vi "Axsun_module.vi"() -> ()   [LabVIEW 2018]
uses:
  cluster_Axsun.ctl
  Queue Manager Actions.ctl
  MessagePacket.ctl
  QueueNames.ctl
  C:/AlazarTech/ATS-SDK/7.2.0/Samples_LabVIEW/ATS9350/Dual Port/stephan/AxsunOCTControl.dll
  AxsunOCTControl.dll
panel:
  in  "clock delay":u32
  in  "GetStatus":bool
  in  "LaserOnTime":bool
  out "output cluster":T1
  out "GUI error":errorcluster
  in  "Source current OFF":bool
  in  "Source current ON":bool
  in  "stop":bool
  in  "Laser OFF":bool
  in  "Laser ON":bool
  out "processor error":errorcluster
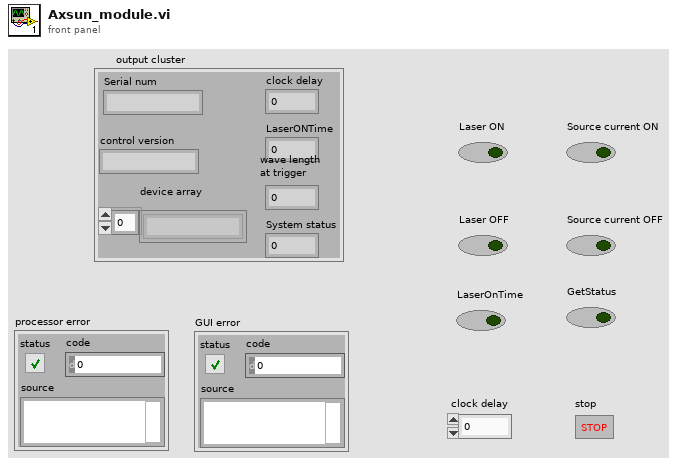
[diagram p1: front panel]
types:
  T1 = typedef "cluster_Axsun.ctl" = cluster{"device array":string[], "control version":string, "Serial num":string, "LaserONTime":i32, "wave length\nat trigger":dbl, "System status":dbl, "clock delay":u32}
  T2 = typedef "MessagePacket.ctl" = cluster{"Message":string, "Parameter":variant}
  T3 = typedef "Queue Manager Actions.ctl" = enum16{"Init", "Enqueue", "Enqueue All", "Preview Queue", "Dequeue", "Get Status", "Flush Queue", "Flush All Queues", "Release All Queues", "Release Queue", "Enqueue at Opposite End"}
  T4 = typedef "QueueNames.ctl" = enum16{"Main GUI", "Main Scan Processor", "Axsun GUI", "Axsun processor", "Main Display", "Main Table Stage GUI", "Main Table Stage Proc.", "Scan Engine", "Vibratome GUI", "Vibratome Processor", "Slice Engine"}
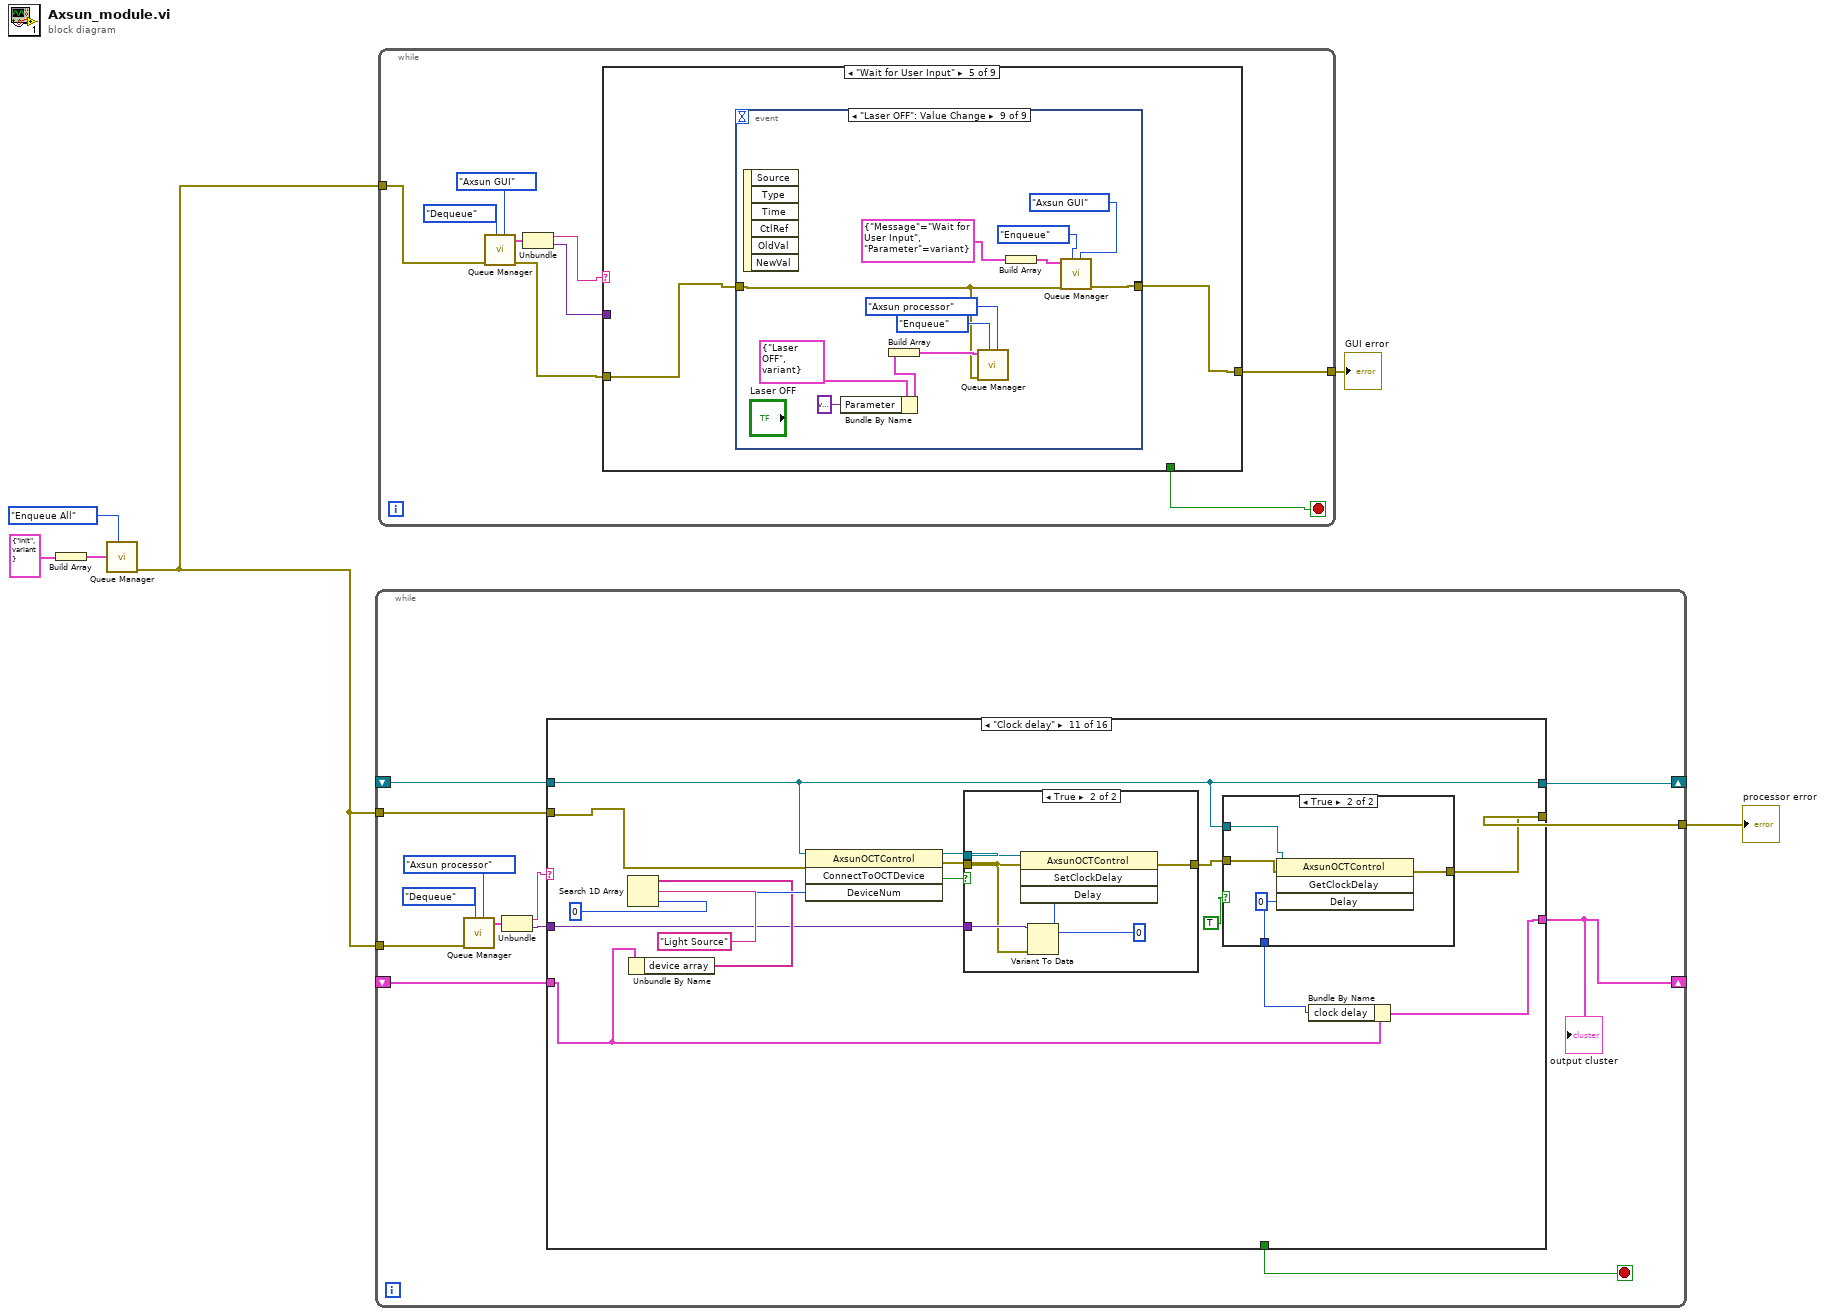
[diagram p0: block diagram]
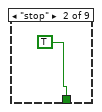
[diagram p3: hidden frame]
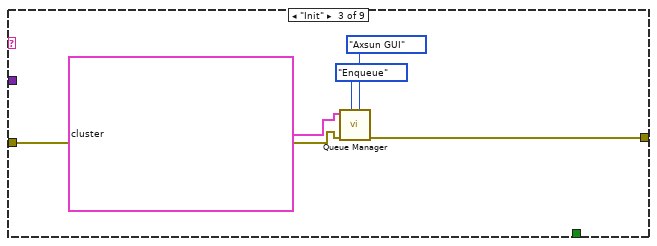
[diagram p4: hidden frame]
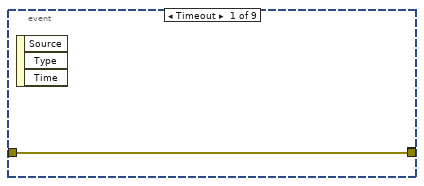
[diagram p6: hidden frame]
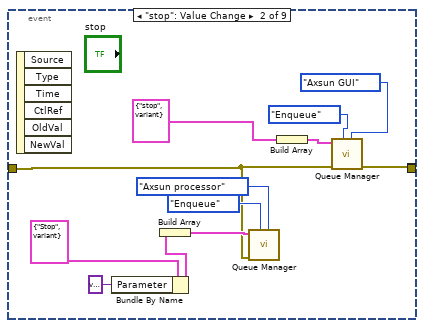
[diagram p7: hidden frame]
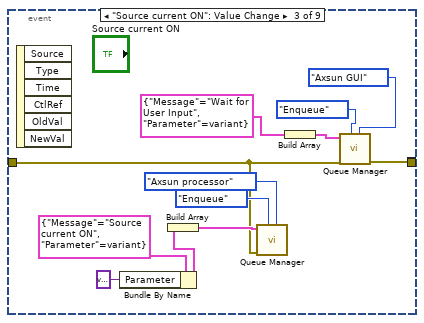
[diagram p8: hidden frame]
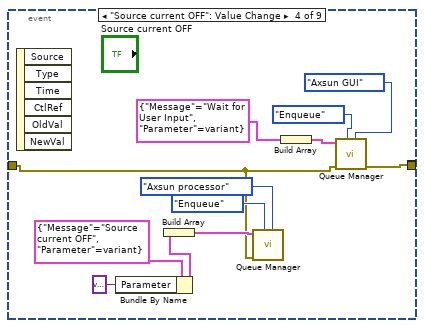
[diagram p9: hidden frame]
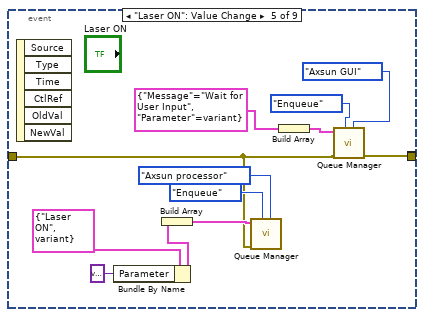
[diagram p10: hidden frame]
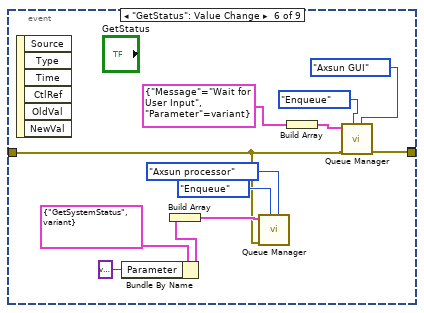
[diagram p11: hidden frame]
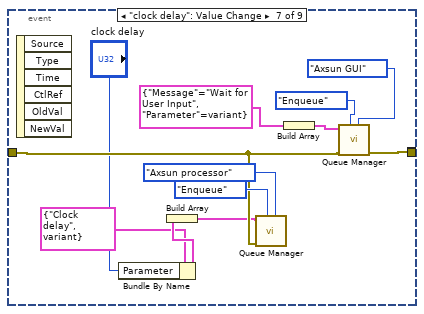
[diagram p12: hidden frame]
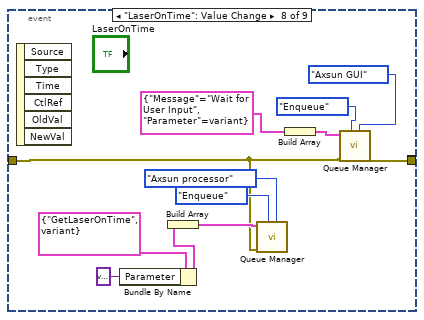
[diagram p13: hidden frame]
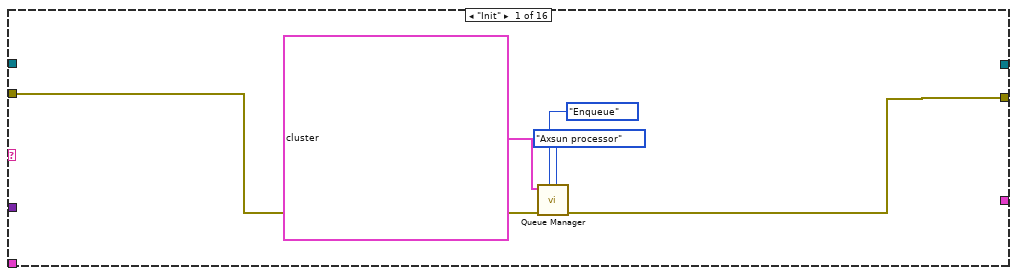
[diagram p18: hidden frame]
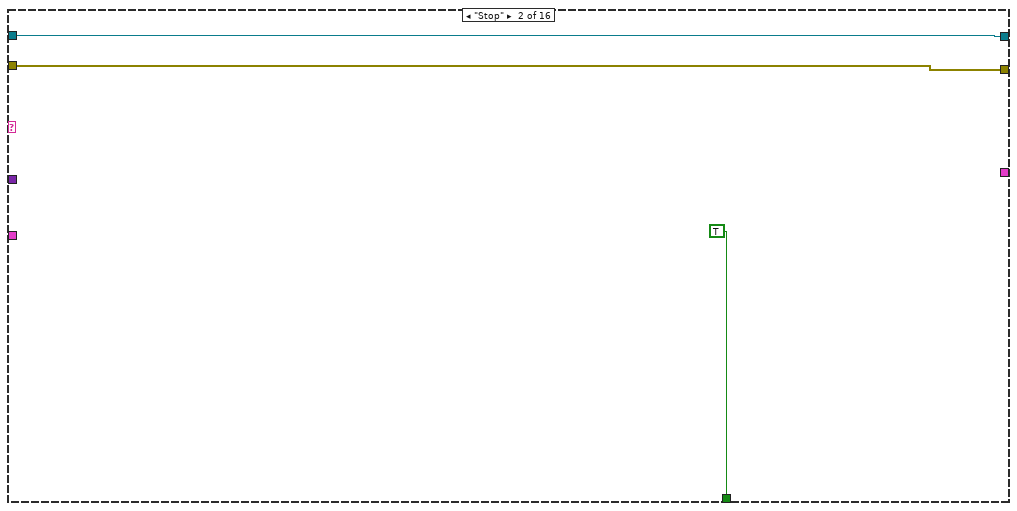
[diagram p19: hidden frame]
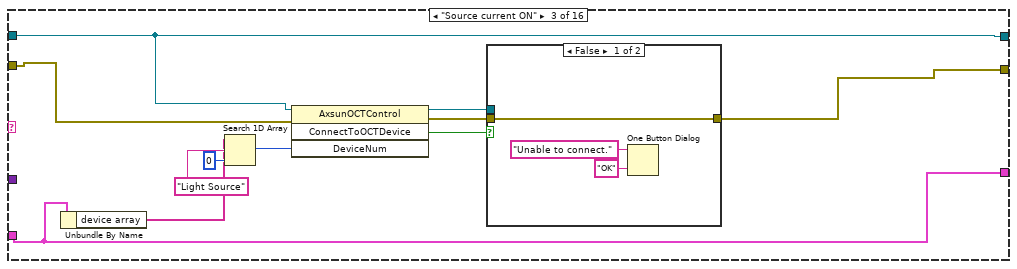
[diagram p20: hidden frame]
diagram:
  n1 = Build Array(T2 {"Message"="Init", "Parameter"=variant} ("Message Packet [In]")) -> (w4:T2[])
  n2 = call "Queue Manager.vi"("Action"=Queue_Manager_Actions."Enqueue All", "Message Packet Array"=w4) -> ("Error Out"=w2:errorcluster)  [unwired: 7 in, 2 out]
  n3 = while {
    shift-right: [w7] -> _
    shift-left: _ -> [w8]
    tunnel: w2 -> [w15]
    shift-right: [w9] -> _
    shift-left: _ -> [w12]
    tunnel: [w11] -> w3
    tunnel: w2 -> [w10]
    stop <- w14 stop-if-true
    n4 = call "Queue Manager.vi"("Queue Name"=QueueNames."Axsun processor", "Action"=Queue_Manager_Actions."Dequeue", "Error In"=w10) -> ("Message Packet [Out]"=w17:T2)  [unwired: 6 in, 2 out]
    n5 = Unbundle(w17) -> ("Message"=w13:string, "Parameter"=w16:variant)
    n6 = case shown="\"Clock delay\"" w13 {
      tunnel: w16 -> [_ _ _ _ _ _ _ _ _ _ w168 _ _ _ _ _]
      tunnel: w15 -> [w24 w26 w32 w48 w64 w69 w86 w106 w125 w146 w169 w198 w216 w223 w244 _]
      tunnel: [_ TRUE _ _ _ _ _ _ _ _ _ _ _ _ _ _] -> w14
      tunnel: [w20 w26 w31 w49 w64 w67 w82 w105 w124 w145 w165 w197 w215 w222 w243 w261] -> w11
      tunnel: [_ _ w30 w47 w63 w66 w75 w104 w123 w143 w163 w196 w213 w218 w240 w260] -> w9
      tunnel: w12 -> [_ _ w30 w47 w63 w66 _ w104 w121 w142 w164 w196 w214 w220 w241 w260]
      tunnel: [_ w25 w28 w45 w62 w65 w72 w102 w119 w140 w161 w194 w211 w217 w239 w259] -> w7
      tunnel: w8 -> [_ w25 w28 w45 w62 w65 w72 w102 w119 w140 w161 w194 w211 w217 w239 _]
      frame "Init" {
        n7 = call "Queue Manager.vi"("Queue Name"=QueueNames."Axsun processor", "Action"=Queue_Manager_Actions."Enqueue", "Error In"=w24, "Message Packet Array"=T2[] [{"Message"="Create handle", "Parameter"=variant}, {"Message"="Start Network Control Interface", "Parameter"=variant}, {"Message"="Get laser handle", "Parameter"=variant}, {"Message"="GetControlVersion", "Parameter"=variant}, {"Message"="GetSerialNum", "Parameter"=variant}, {"Message"="GetSystemStatus", "Parameter"=variant}, {"Message"="GetWaveLengthAtSweptTrigger", "Parameter"=variant}, {"Message"="GetLaserOnTime\nGetLaserOnTime", "Parameter"=variant}]) -> ("Error Out"=w20:errorcluster)  [unwired: 5 in, 2 out]
      }
      frame "Stop" {
      }
      frame "Source current ON" {
        n8 = Unbundle By Name(w30) -> ("device array"=w29:string[])
        n9 = Search 1D Array(1D array=w29, element="Light Source", start index (0)=0) -> (index of element=w36:i32)
        n10 = invoke class="AxsunOCTControl" method="ConnectToOCTDevice"(reference=w28, error in=w32, "DeviceNum"=w36) -> (reference out=w35:refnum<k24>, error out=w34:errorcluster, "ConnectToOCTDevice"=w33:bool)  [unwired: 1 in, 1 out]
        n11 = case shown="False" w33 {
          tunnel: w35 -> [_ w44]
          tunnel: w34 -> [w41 w43]
          tunnel: [w41 w42] -> w31
          frame False {
            n12 = One Button Dialog(message="Unable to connect.", button name ("OK")="OK") -> ()  [unwired: 1 out]
          }
          frame True {
            n13 = invoke class="AxsunOCTControl" method="SourceCurrentOn"(reference=w44, error in=w43) -> (error out=w42:errorcluster)  [unwired: 1 in, 2 out]
          }
        }
      }
      frame "Source current OFF" {
        n14 = Unbundle By Name(w47) -> ("device array"=w46:string[])
        n15 = Search 1D Array(1D array=w46, element="Light Source", start index (0)=0) -> (index of element=w53:i32)
        n16 = invoke class="AxsunOCTControl" method="ConnectToOCTDevice"(reference=w45, error in=w48, "DeviceNum"=w53) -> (reference out=w52:refnum<k24>, error out=w51:errorcluster, "ConnectToOCTDevice"=w50:bool)  [unwired: 1 in, 1 out]
        n17 = case shown="True" w50 {
          tunnel: w52 -> [_ w61]
          tunnel: w51 -> [w58 w60]
          tunnel: [w58 w59] -> w49
          frame False {
            n18 = One Button Dialog(message="Unable to connect.", button name ("OK")="OK") -> ()  [unwired: 1 out]
          }
          frame True {
            # "Turn laser emission ON"
            n19 = invoke class="AxsunOCTControl" method="SourceCurrentOff"(reference=w61, error in=w60) -> (error out=w59:errorcluster)  [unwired: 1 in, 2 out]
          }
        }
      }
      frame Default {
      }
      frame "Start Network Control Interface" {
        n20 = invoke class="AxsunOCTControl" method="StartNetworkControlInterface"(reference=w65, error in=w69) -> (error out=w68:errorcluster)  [unwired: 1 in, 2 out]
        n21 = flat-sequence {
          tunnel: w68 -> [w70]
          tunnel: [w70] -> w67
          frame #0 {
            n22 = Wait (ms)(milliseconds to wait=2000) -> ()  [unwired: 1 out]
          }
        }
      }
      frame "Get laser handle" {
        n23 = invoke class="AxsunOCTControl" method="GetNumberOfOCTDevicesPresent"(reference=w72, error in=w86) -> (reference out=w85:refnum<k24>, error out=w83:errorcluster, "GetNumberOfOCTDevicesPresent"=w84:i32)  [unwired: 1 in]
        n24 = for {
          N: w84 -> [_]
          tunnel: w85 -> [w92]
          tunnel: w83 -> [w91]
          tunnel: [w87] -> w77 mode=indexing
          tunnel: [w89] -> w82
          tunnel: [w88] -> _ mode=indexing
          i -> [w90]
          n25 = invoke class="AxsunOCTControl" method="ConnectToOCTDevice"(reference=w92, error in=w91, "DeviceNum"=w90) -> (reference out=w96:refnum<k24>, error out=w95:errorcluster)  [unwired: 1 in, 2 out]
          n26 = stacked-sequence {
            tunnel: w96 -> [w101]
            tunnel: [w101] -> w94
            tunnel: w95 -> [w100]
            tunnel: [w100] -> w93
            frame #0 {
              n27 = Wait (ms)(milliseconds to wait=u32 20) -> ()  [unwired: 1 out]
            }
          }
          n28 = invoke class="AxsunOCTControl" method="GetSystemType"(reference=w94, error in=w93, "SystemType"=u32 0, "SystemTypeString"="") -> (reference out=w88:refnum<k24>, error out=w89:errorcluster, "SystemTypeString"=w87:string)  [unwired: 1 in, 2 out]
        }
        n29 = Bundle By Name(cluster=T1 {"device array"=[], "control version"="", "Serial num"="", "LaserONTime"=0, "wave length\nat trigger"=0.0, "System status"=0.0, "clock delay"=0} ("output cluster"), "device array"=w77, "control version"="GetControlVersion", "Serial num"="''", "LaserONTime"=0, "wave length\nat trigger"=0.0, "System status"=0.0 ("Status"), "clock delay"=u32 0) -> (w75:T1)
      }
      frame "Laser ON" {
        n30 = Unbundle By Name(w104) -> ("device array"=w103:string[])
        n31 = Search 1D Array(1D array=w103, element="Light Source", start index (0)=0) -> (index of element=w110:i32)
        n32 = invoke class="AxsunOCTControl" method="ConnectToOCTDevice"(reference=w102, error in=w106, "DeviceNum"=w110) -> (reference out=w109:refnum<k24>, error out=w108:errorcluster, "ConnectToOCTDevice"=w107:bool)  [unwired: 1 in, 1 out]
        n33 = case shown="True" w107 {
          tunnel: w109 -> [_ w118]
          tunnel: w108 -> [w115 w117]
          tunnel: [w115 w116] -> w105
          frame False {
            n34 = One Button Dialog(message="Unable to .", button name ("OK")="OK") -> ()  [unwired: 1 out]
          }
          frame True {
            # "Turn laser emission ON"
            n35 = invoke class="AxsunOCTControl" method="StartScan"(reference=w118, error in=w117) -> (error out=w116:errorcluster)  [unwired: 1 in, 2 out]
          }
        }
      }
      frame "GetWaveLengthAtSweptTrigger" {
        n36 = Unbundle By Name(w121) -> ("device array"=w120:string[])
        n37 = Search 1D Array(1D array=w120, element="Light Source", start index (0)=0) -> (index of element=w129:i32)
        n38 = invoke class="AxsunOCTControl" method="ConnectToOCTDevice"(reference=w119, error in=w125, "DeviceNum"=w129) -> (reference out=w128:refnum<k24>, error out=w127:errorcluster, "ConnectToOCTDevice"=w126:bool)  [unwired: 1 in, 1 out]
        n39 = case shown="False" w126 {
          tunnel: w128 -> [_ w139]
          tunnel: w127 -> [w134 w138]
          tunnel: [w134 w137] -> w124
          tunnel: [_ w135] -> w122
          frame False {
            n40 = One Button Dialog(message="Unable to .", button name ("OK")="OK") -> ()  [unwired: 1 out]
          }
          frame True {
            # "Turn laser emission ON"
            n41 = invoke class="AxsunOCTControl" method="GetWavelengthAtSweepTrigger"(reference=w139, error in=w138, "Wavelength"=0.0) -> (error out=w137:errorcluster, "Wavelength"=w135:dbl)  [unwired: 1 in, 2 out]
          }
        }
        n42 = Bundle(cluster=w121, "LaserONTime"=w122) -> (w123:T1)  [unwired: 6 in]
      }
      frame "GetLaserOnTime" {
        # "Make active board = laser"
        n43 = Unbundle By Name(w142) -> ("device array"=w141:string[])
        n44 = Search 1D Array(1D array=w141, element="Light Source", start index (0)=0) -> (index of element=w152:i32)
        n45 = invoke class="AxsunOCTControl" method="ConnectToOCTDevice"(reference=w140, error in=w146, "DeviceNum"=w152) -> (reference out=w148:refnum<k24>, error out=w149:errorcluster, "ConnectToOCTDevice"=w147:bool)  [unwired: 1 in, 1 out]
        n46 = case shown="False" w147 {
          tunnel: w149 -> [w155 w159]
          tunnel: w148 -> [_ w160]
          tunnel: [w155 w158] -> w145
          tunnel: [_ w156] -> w144
          frame False {
            n47 = One Button Dialog(message="Unable to connect.", button name ("OK")="OK") -> ()  [unwired: 1 out]
          }
          frame True {
            n48 = invoke class="AxsunOCTControl" method="GetLaserOnTime"(reference=w160, error in=w159, "LaserOnTimeSeconds"=u32 0) -> (error out=w158:errorcluster, "LaserOnTimeSeconds"=w156:u32)  [unwired: 1 in, 2 out]
          }
        }
        n49 = Bundle(cluster=w142, "LaserONTime"=w144) -> (w143:T1)  [unwired: 6 in]
      }
      frame "Clock delay" {
        n50 = Unbundle By Name(w164) -> ("device array"=w170:string[])
        n51 = Search 1D Array(1D array=w170, element="Light Source", start index (0)=0) -> (index of element=w174:i32)
        n52 = invoke class="AxsunOCTControl" method="ConnectToOCTDevice"(reference=w161, error in=w169, "DeviceNum"=w174) -> (reference out=w173:refnum<k24>, error out=w172:errorcluster, "ConnectToOCTDevice"=w171:bool)  [unwired: 1 in, 1 out]
        n53 = case shown="True" w171 {
          tunnel: w173 -> [_ w193]
          tunnel: w172 -> [w187 w189]
          tunnel: [w187 w188] -> w167
          tunnel: w168 -> [_ w192]
          frame False {
            n54 = One Button Dialog(message="Unable to connect.", button name ("OK")="OK") -> ()  [unwired: 1 out]
          }
          frame True {
            n55 = Variant To Data(error in=w189, type=u32 0 ("Delay"), Variant=w192) -> (data=w190:u32)  [unwired: 1 out]
            n56 = invoke class="AxsunOCTControl" method="SetClockDelay"(reference=w193, error in=w189, "Delay"=w190) -> (error out=w188:errorcluster)  [unwired: 1 in, 3 out]
          }
        }
        n57 = case shown="True" TRUE {
          tunnel: w167 -> [w179 w184]
          tunnel: [w179 w183] -> w165
          tunnel: [_ w181] -> w162
          tunnel: w161 -> [_ w180]
          frame False {
            n58 = One Button Dialog(message="Unable to connect.", button name ("OK")="OK") -> ()  [unwired: 1 out]
          }
          frame True {
            n59 = invoke class="AxsunOCTControl" method="GetClockDelay"(reference=w180, error in=w184, "Delay"=u32 0) -> (error out=w183:errorcluster, "Delay"=w181:u32)  [unwired: 1 in, 2 out]
          }
        }
        n60 = Bundle By Name(cluster=w164, "clock delay"=w162) -> (w163:T1)
      }
      frame "Laser OFF" {
        # "Make active board = laser"
        n61 = Unbundle By Name(w196) -> ("device array"=w195:string[])
        n62 = Search 1D Array(1D array=w195, element="Light Source", start index (0)=0) -> (index of element=w202:i32)
        n63 = invoke class="AxsunOCTControl" method="ConnectToOCTDevice"(reference=w194, error in=w198, "DeviceNum"=w202) -> (reference out=w201:refnum<k24>, error out=w200:errorcluster, "ConnectToOCTDevice"=w199:bool)  [unwired: 1 in, 1 out]
        n64 = case shown="True" w199 {
          tunnel: w201 -> [_ w210]
          tunnel: w200 -> [w207 w209]
          tunnel: [w207 w208] -> w197
          frame False {
            n65 = One Button Dialog(message="Unable to connect.", button name ("OK")="OK") -> ()  [unwired: 1 out]
          }
          frame True {
            # "Turn laser emission ON"
            n66 = invoke class="AxsunOCTControl" method="StopScan"(reference=w210, error in=w209) -> (error out=w208:errorcluster)  [unwired: 1 in, 2 out]
          }
        }
      }
      frame "GetControlVersion" {
        n67 = invoke class="AxsunOCTControl" method="GetControlVersion"(reference=w211, error in=w216) -> (error out=w215:errorcluster, "GetControlVersion"=w212:string)  [unwired: 1 in, 1 out]
        n68 = Bundle By Name(cluster=w214, "control version"=w212) -> (w213:T1)
      }
      frame "GetSerialNum" {
        n69 = Unbundle By Name(w220) -> ("device array"=w221:string[])
        n70 = Search 1D Array(1D array=w221, element="Light Source", start index (0)=0) -> (index of element=w227:i32)
        n71 = invoke class="AxsunOCTControl" method="ConnectToOCTDevice"(reference=w217, error in=w223, "DeviceNum"=w227) -> (reference out=w226:refnum<k24>, error out=w225:errorcluster, "ConnectToOCTDevice"=w224:bool)  [unwired: 1 in, 1 out]
        n72 = case shown="True" w224 {
          tunnel: w226 -> [_ w237]
          tunnel: w225 -> [w232 w236]
          tunnel: [w232 w235] -> w222
          tunnel: [_ w233] -> w219
          frame False {
            n73 = One Button Dialog(message="Unable to connect.", button name ("OK")="OK") -> ()  [unwired: 1 out]
          }
          frame True {
            n74 = invoke class="AxsunOCTControl" method="GetSerialNum"(reference=w237, error in=w236, "SerialNum"="") -> (error out=w235:errorcluster, "SerialNum"=w233:string)  [unwired: 1 in, 2 out]
          }
        }
        n75 = Bundle By Name(cluster=w220, "Serial num"=w219) -> (w218:T1)
      }
      frame "GetSystemStatus" {
        # "Make active board = laser"
        n76 = Unbundle By Name(w241) -> ("device array"=w242:string[])
        n77 = Search 1D Array(1D array=w242, element="Light Source", start index (0)=0) -> (index of element=w249:i32)
        n78 = invoke class="AxsunOCTControl" method="ConnectToOCTDevice"(reference=w239, error in=w244, "DeviceNum"=w249) -> (error out=w245:errorcluster, "ConnectToOCTDevice"=w246:bool)  [unwired: 1 in, 2 out]
        n79 = case shown="True" w246 {
          tunnel: w245 -> [w252 w258]
          tunnel: [w252 w255] -> w243
          tunnel: [_ w254] -> w238
          tunnel: w239 -> [_ w253]
          frame False {
            n80 = One Button Dialog(message="Unable to connect.", button name ("OK")="OK") -> ()  [unwired: 1 out]
          }
          frame True {
            n81 = invoke class="AxsunOCTControl" method="GetSystemStatus"(reference=w253, error in=w258, "StatusArray"=u32[] [], "StatusWordsReturned"=u32 0) -> (error out=w255:errorcluster, "StatusWordsReturned"=w254:u32)  [unwired: 1 in, 3 out]
          }
        }
        n82 = Bundle By Name(cluster=w241, "System status"=w238) -> (w240:T1)
      }
      frame "Create handle" {
        n83 = constructor class="AxsunOCTControl"() -> (reference out=w259:refnum<k24>, error out=w261:errorcluster)  [unwired: 3 in, 1 out]
      }
    }
    "output cluster" <- w9
  }
  "processor error" <- w3
  n84 = while {
    tunnel: w2 -> [w267]
    tunnel: [w263] -> w1
    stop <- w262 stop-if-true
    n85 = call "Queue Manager.vi"("Queue Name"=QueueNames."Axsun GUI", "Action"=Queue_Manager_Actions."Dequeue", "Error In"=w267) -> ("Error Out"=w264:errorcluster, "Message Packet [Out]"=w268:T2)  [unwired: 6 in, 1 out]
    n86 = Unbundle(w268) -> ("Message"=w266:string, "Parameter"=w265:variant)
    n87 = case shown="\"Wait for User Input\"" w266 {
      tunnel: w265 -> [_ _ _ _ _ _ _ _ _]
      tunnel: w264 -> [w271 _ w277 w278 w280 w378 w379 w380 w381]
      tunnel: [w271 _ w274 w278 w279 w378 w379 w380 w381] -> w263
      tunnel: [_ TRUE _ _ _ _ _ _ _] -> w262
      frame "False", Default {
      }
      frame "stop" {
      }
      frame "Init" {
        n88 = call "Queue Manager.vi"("Queue Name"=QueueNames."Axsun GUI", "Action"=Queue_Manager_Actions."Enqueue", "Error In"=w277, "Message Packet Array"=T2[] [{"Message"="Wait for Complete", "Parameter"=variant}, {"Message"="Set Front Panel", "Parameter"=variant}, {"Message"="Load User Settings", "Parameter"=variant}, {"Message"="Configure Hardware", "Parameter"=variant}, {"Message"="Configure Hardware", "Parameter"=variant}, {"Message"="Wait for User Input", "Parameter"=variant}]) -> ("Error Out"=w274:errorcluster)  [unwired: 5 in, 2 out]
      }
      frame "Set Front Panel" {
      }
      frame "Wait for User Input" {
        n89 = event shown="[8] \"Laser OFF\": Value Change" {
          selector: _ -> [_ _ _ _ _ _ _ _ _]
          dyn-events: _ -> [_ _ _ _ _ _ _ _ _]
          timeout: _ -> [_ _ _ _ _ _ _ _ _]
          tunnel: w280 -> [w281 w282 w294 w306 w318 w331 w346 w355 w366]
          tunnel: [_ w283 w295 w307 w322 w330 w345 w354 w368] -> w279
          tunnel: [w281 _ _ _ _ _ _ _ _] -> _
          event Timeout {
            n90 = event-data() -> ()  [unwired: 1 in, 3 out]
          }
          event "stop": Value Change {
            n91 = event-data() -> ()  [unwired: 1 in, 6 out]
            n92 = Bundle By Name(cluster=T2 {"Message"="Stop", "Parameter"=variant} ("Message Packet [In]"), "Parameter"=variant) -> (w289:T2)
            n93 = Build Array(w289) -> (w286:T2[])
            n94 = call "Queue Manager.vi"("Queue Name"=QueueNames."Axsun processor", "Action"=Queue_Manager_Actions."Enqueue", "Error In"=w282, "Message Packet Array"=w286) -> ()  [unwired: 5 in, 3 out]
            n95 = Build Array(T2 {"Message"="stop", "Parameter"=variant} ("Message Packet [In]")) -> (w293:T2[])
            n96 = call "Queue Manager.vi"("Queue Name"=QueueNames."Axsun GUI", "Action"=Queue_Manager_Actions."Enqueue", "Error In"=w282, "Message Packet Array"=w293) -> ("Error Out"=w283:errorcluster)  [unwired: 5 in, 2 out]
          }
          event "Source current ON": Value Change {
            n97 = event-data() -> ()  [unwired: 1 in, 6 out]
            n98 = Bundle By Name(cluster=T2 {"Message"="Source current ON", "Parameter"=variant} ("Message Packet [In]"), "Parameter"=variant) -> (w301:T2)
            n99 = Build Array(w301) -> (w298:T2[])
            n100 = call "Queue Manager.vi"("Queue Name"=QueueNames."Axsun processor", "Action"=Queue_Manager_Actions."Enqueue", "Error In"=w294, "Message Packet Array"=w298) -> ()  [unwired: 5 in, 3 out]
            n101 = Build Array(T2 {"Message"="Wait for User Input", "Parameter"=variant} ("Message Packet [In]")) -> (w305:T2[])
            n102 = call "Queue Manager.vi"("Queue Name"=QueueNames."Axsun GUI", "Action"=Queue_Manager_Actions."Enqueue", "Error In"=w294, "Message Packet Array"=w305) -> ("Error Out"=w295:errorcluster)  [unwired: 5 in, 2 out]
          }
          event "Source current OFF": Value Change {
            n103 = event-data() -> ()  [unwired: 1 in, 6 out]
            n104 = Bundle By Name(cluster=T2 {"Message"="Source current OFF", "Parameter"=variant} ("Message Packet [In]"), "Parameter"=variant) -> (w313:T2)
            n105 = Build Array(w313) -> (w310:T2[])
            n106 = call "Queue Manager.vi"("Queue Name"=QueueNames."Axsun processor", "Action"=Queue_Manager_Actions."Enqueue", "Error In"=w306, "Message Packet Array"=w310) -> ()  [unwired: 5 in, 3 out]
            n107 = Build Array(T2 {"Message"="Wait for User Input", "Parameter"=variant} ("Message Packet [In]")) -> (w317:T2[])
            n108 = call "Queue Manager.vi"("Queue Name"=QueueNames."Axsun GUI", "Action"=Queue_Manager_Actions."Enqueue", "Error In"=w306, "Message Packet Array"=w317) -> ("Error Out"=w307:errorcluster)  [unwired: 5 in, 2 out]
          }
          event "Laser ON": Value Change {
            n109 = event-data() -> ()  [unwired: 1 in, 6 out]
            n110 = Bundle By Name(cluster=T2 {"Message"="Laser ON", "Parameter"=variant} ("Message Packet [In]"), "Parameter"=variant) -> (w325:T2)
            n111 = Build Array(w325) -> (w321:T2[])
            n112 = call "Queue Manager.vi"("Queue Name"=QueueNames."Axsun processor", "Action"=Queue_Manager_Actions."Enqueue", "Error In"=w318, "Message Packet Array"=w321) -> ()  [unwired: 5 in, 3 out]
            n113 = Build Array(T2 {"Message"="Wait for User Input", "Parameter"=variant} ("Message Packet [In]")) -> (w329:T2[])
            n114 = call "Queue Manager.vi"("Queue Name"=QueueNames."Axsun GUI", "Action"=Queue_Manager_Actions."Enqueue", "Error In"=w318, "Message Packet Array"=w329) -> ("Error Out"=w322:errorcluster)  [unwired: 5 in, 2 out]
          }
          event "GetStatus": Value Change {
            n115 = event-data() -> ()  [unwired: 1 in, 6 out]
            n116 = Bundle By Name(cluster=T2 {"Message"="GetSystemStatus", "Parameter"=variant} ("Message Packet [In]"), "Parameter"=variant) -> (w337:T2)
            n117 = Build Array(w337) -> (w334:T2[])
            n118 = call "Queue Manager.vi"("Queue Name"=QueueNames."Axsun processor", "Action"=Queue_Manager_Actions."Enqueue", "Error In"=w331, "Message Packet Array"=w334) -> ()  [unwired: 5 in, 3 out]
            n119 = Build Array(T2 {"Message"="Wait for User Input", "Parameter"=variant} ("Message Packet [In]")) -> (w341:T2[])
            n120 = call "Queue Manager.vi"("Queue Name"=QueueNames."Axsun GUI", "Action"=Queue_Manager_Actions."Enqueue", "Error In"=w331, "Message Packet Array"=w341) -> ("Error Out"=w330:errorcluster)  [unwired: 5 in, 2 out]
          }
          event "clock delay": Value Change {
            n121 = event-data() -> ()  [unwired: 1 in, 6 out]
            n122 = Bundle By Name(cluster=T2 {"Message"="Clock delay", "Parameter"=variant} ("Message Packet [In]"), "Parameter"="clock delay") -> (w349:T2)
            n123 = Build Array(w349) -> (w343:T2[])
            n124 = call "Queue Manager.vi"("Queue Name"=QueueNames."Axsun processor", "Action"=Queue_Manager_Actions."Enqueue", "Error In"=w346, "Message Packet Array"=w343) -> ()  [unwired: 5 in, 3 out]
            n125 = Build Array(T2 {"Message"="Wait for User Input", "Parameter"=variant} ("Message Packet [In]")) -> (w353:T2[])
            n126 = call "Queue Manager.vi"("Queue Name"=QueueNames."Axsun GUI", "Action"=Queue_Manager_Actions."Enqueue", "Error In"=w346, "Message Packet Array"=w353) -> ("Error Out"=w345:errorcluster)  [unwired: 5 in, 2 out]
          }
          event "LaserOnTime": Value Change {
            n127 = event-data() -> ()  [unwired: 1 in, 6 out]
            n128 = Bundle By Name(cluster=T2 {"Message"="GetLaserOnTime", "Parameter"=variant} ("Message Packet [In]"), "Parameter"=variant) -> (w361:T2)
            n129 = Build Array(w361) -> (w358:T2[])
            n130 = call "Queue Manager.vi"("Queue Name"=QueueNames."Axsun processor", "Action"=Queue_Manager_Actions."Enqueue", "Error In"=w355, "Message Packet Array"=w358) -> ()  [unwired: 5 in, 3 out]
            n131 = Build Array(T2 {"Message"="Wait for User Input", "Parameter"=variant} ("Message Packet [In]")) -> (w365:T2[])
            n132 = call "Queue Manager.vi"("Queue Name"=QueueNames."Axsun GUI", "Action"=Queue_Manager_Actions."Enqueue", "Error In"=w355, "Message Packet Array"=w365) -> ("Error Out"=w354:errorcluster)  [unwired: 5 in, 2 out]
          }
          event "Laser OFF": Value Change {
            n133 = event-data() -> ()  [unwired: 1 in, 6 out]
            n134 = Bundle By Name(cluster=T2 {"Message"="Laser OFF", "Parameter"=variant} ("Message Packet [In]"), "Parameter"=variant) -> (w373:T2)
            n135 = Build Array(w373) -> (w370:T2[])
            n136 = call "Queue Manager.vi"("Queue Name"=QueueNames."Axsun processor", "Action"=Queue_Manager_Actions."Enqueue", "Error In"=w366, "Message Packet Array"=w370) -> ()  [unwired: 5 in, 3 out]
            n137 = Build Array(T2 {"Message"="Wait for User Input", "Parameter"=variant} ("Message Packet [In]")) -> (w377:T2[])
            n138 = call "Queue Manager.vi"("Queue Name"=QueueNames."Axsun GUI", "Action"=Queue_Manager_Actions."Enqueue", "Error In"=w366, "Message Packet Array"=w377) -> ("Error Out"=w368:errorcluster)  [unwired: 5 in, 2 out]
          }
        }
      }
      frame "Wait for Complete" {
      }
      frame "Configure Hardware" {
      }
      frame "Load User Settings" {
      }
      frame "Init Variables" {
      }
    }
  }
  "GUI error" <- w1
